vi "Write Channels.vi"(8 "error in (no error)":errorcluster, 10 "Channels Array":refnum<class "Channel.lvclass">[](array[class]), 11 "Channel Manager in":refnum<class "Channel Manager.lvclass">) -> (0 "error out":errorcluster, 3 "Channel Manager out":refnum<class "Channel Manager.lvclass">)   [LabVIEW 2018, in "Channel Manager.lvclass"]
uses:
  Channel Manager.lvclass
  Channel/Channel.lvclass
  Channel Manager.lvclass/Channel Manager.ctl
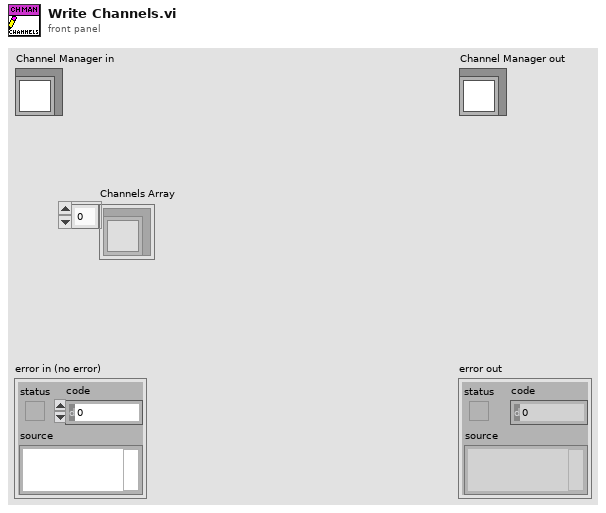
[diagram p1: front panel]
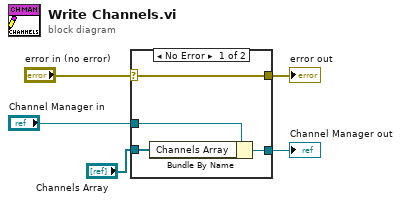
[diagram p0: block diagram]
diagram:
  n1 = case shown="No Error" "error in (no error)" {
    selector: "error in (no error)" -> [w9 w10]
    tunnel: [w9 w10] -> w4
    tunnel: [w6 w11] -> w2
    tunnel: "Channel Manager in" -> [w8 w11]
    tunnel: "Channels Array" -> [w7 _]
    frame No Error {
      n2 = Bundle By Name(cluster=w8, "Channels Array"=w7) -> (w6:refnum<class "Channel Manager.lvclass">)
    }
    frame Error {
    }
  }
  "error out" <- w4
  "Channel Manager out" <- w2
